vi "Stream-to-file.vi"(8 "error in (no error)":errorcluster, 11 "Errors in":T1) -> (0 "error out":errorcluster, 3 "Errors out":T1)   [LabVIEW 2013, in "Error-handling.lvlib" / "Errors.lvclass"]
uses:
  Errors.lvclass
  Object-reference.ctl
  Errors.lvclass/Errors.ctl
  <vilib>/Utility/error.llb/DialogType.ctl
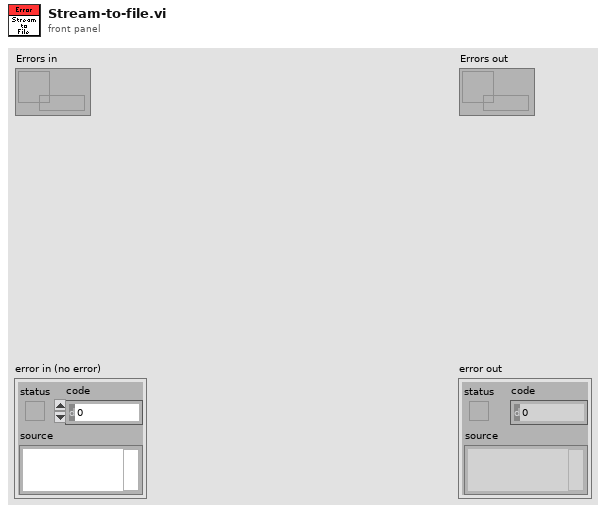
[diagram p1: front panel]
types:
  T1 = typedef "Error-handling.lvlib/Errors.lvclass/Object-reference.ctl" = refnum<data-value>
  T2 = typedef "DialogType.ctl" = u16
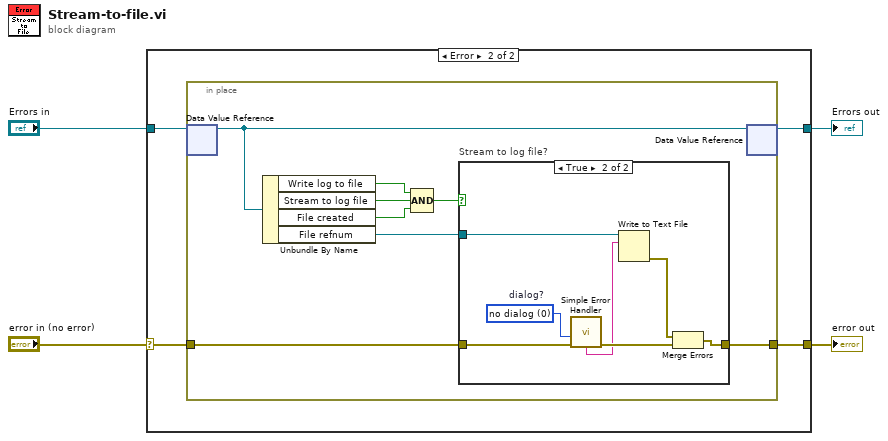
[diagram p0: block diagram]
diagram:
  n1 = case shown="Error" "error in (no error)" {
    selector: "error in (no error)" -> [w6 w10]
    tunnel: [w6 w9] -> w3
    tunnel: [w5 w7] -> w1
    tunnel: "Errors in" -> [w5 w8]
    frame No Error {
    }
    frame Error {
      n2 = in-place {
        in-place-border: w10 -> [w16]
        in-place-border: [w15] -> w9
        n3 = in-place-dvr #1(w8) -> (w11:refnum<class "Errors.lvclass">)  [unwired: 1 out]
        n4 = Unbundle By Name(w11) -> ("Write log to file"=w12:bool, "Stream to log file"=w13:bool, "File created"=w14:bool, "File refnum"=w17:refnum<file>)
        n5 = Compound Arithmetic op=AND(w12, w13, w14) -> (w18:bool)
        n6 = case "Stream to log file?" shown="True" w18 {
          tunnel: w17 -> [_ w26]
          tunnel: w16 -> [w19 w24]
          tunnel: [w19 w22] -> w15
          frame False {
          }
          frame True {
            w25 = T2 0 items=["no dialog", "OK message", "continue or stop message", "OK message + warnings", "continue/stop + warnings"]  # dialog?
            n7 = call <vilib>:"Simple Error Handler.vi"("type of dialog (OK msg:1)"=w25, "error in (no error)"=w24) -> ("error out"=w23:errorcluster, "message"=w20:string)  [unwired: 3 in, 3 out]
            n8 = Write to Text File(file (use dialog)=w26, text=w20) -> (error out=w21:errorcluster)  [unwired: 2 in, 2 out]
            n9 = Merge Errors(w21, w23) -> (w22:errorcluster)
          }
        }
        n10 = in-place-dvr #1(w11) -> (w7:T1)  [unwired: 1 out]
      }
    }
  }
  "error out" <- w3
  "Errors out" <- w1
